vi "LED.vi"() -> ()   [LabVIEW 2020]
panel:
  in  "Color 5":u32(colorbox)=15663339
  in  "Color 4":u32(colorbox)=16777215
  in  "Color 3":u32(colorbox)=16711680
  in  "Color 2":u32(colorbox)=65511
  in  "Color":u32(colorbox)=6618880
  out "error out":errorcluster
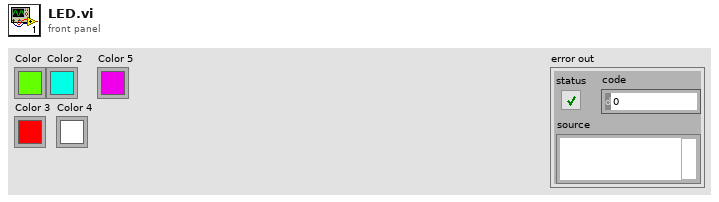
[diagram p1: front panel]
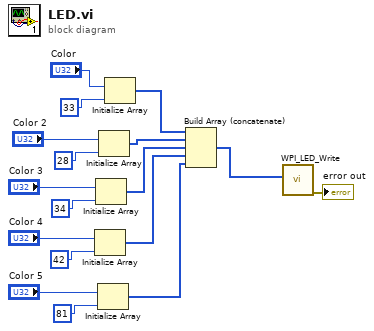
[diagram p0: block diagram]
diagram:
  n1 = Initialize Array("Color 4", 42 ("dimension size")) -> (w2:u32[])
  n2 = Initialize Array("Color 3", 34 ("dimension size")) -> (w7:u32[])
  n3 = Initialize Array("Color 5", 81 ("dimension size")) -> (w1:u32[])
  n4 = Initialize Array("Color 2", 28 ("dimension size")) -> (w10:u32[])
  n5 = Initialize Array("Color", 33 ("dimension size")) -> (w14:u32[])
  n6 = Build Array (concatenate)(w14, w10, w7, w2, w1) -> (w15:u32[])
  n7 = call <vilib>:"WPI_LED_Write.vi"("Color Array"=w15) -> ("error out"=→"error out":errorcluster)  [unwired: 10 in]
